vi "ShowWaveform.vi"(8 "error in (no error)":errorcluster, 10 "Value":waveform(dbl)[](array[waveform]), 11 "NI_DAQmx(AI) in":refnum<class "NI_DAQmx(AI).lvclass">) -> (0 "error out":errorcluster, 3 "NI_DAQmx(AI) out":refnum<class "NI_DAQmx(AI).lvclass">)   [LabVIEW 2025, in "NI_DAQmx(AI).lvclass"]
uses:
  NI_DAQmx(AI).lvclass
  NI_DAQmx(AI).lvclass/NI_DAQmx(AI).ctl
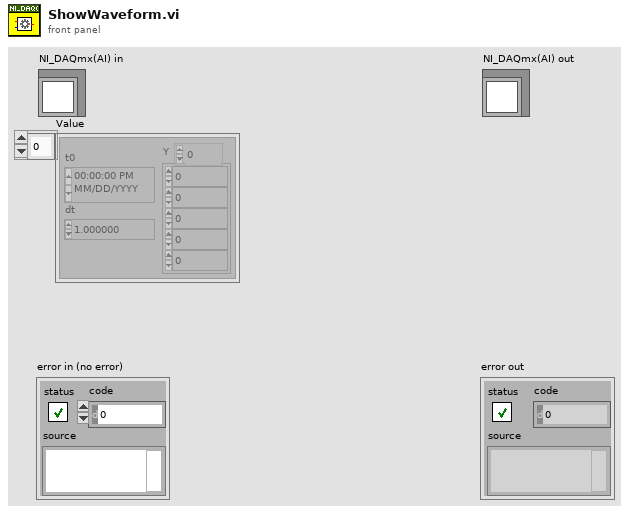
[diagram p1: front panel]
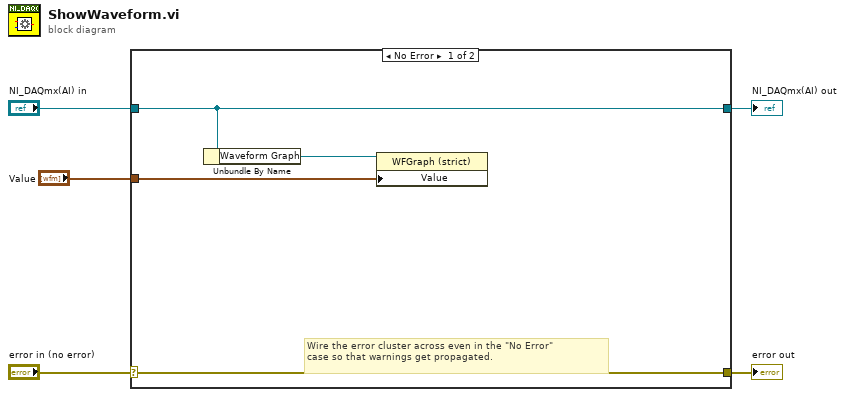
[diagram p0: block diagram]
diagram:
  n1 = case shown="No Error" "error in (no error)" {
    selector: "error in (no error)" -> [w9 w11]
    tunnel: [w9 w11] -> w4
    tunnel: [w8 w10] -> w2
    tunnel: "NI_DAQmx(AI) in" -> [w8 w10]
    tunnel: "Value" -> [w6 _]
    frame No Error {
      # "Wire the error cluster across even in the \"No Error\"\ncase so that warnings get propagated."
      n2 = Unbundle By Name(w8) -> ("Waveform Graph"=w7:refnum<vi>)
      n3 = property class="WFGraph (strict)"(reference=w7, "Value"=w6) -> ()  [unwired: 1 in, 2 out]
    }
    frame Error {
    }
  }
  "error out" <- w4
  "NI_DAQmx(AI) out" <- w2
